vi "INI文件查看器.vi"() -> ()   [LabVIEW 2012, in "Tree Tools.lvlib"]
uses:
  Tree Tools.lvlib
  Core Class/Tree Class/Tree Class.lvclass
  <vilib>/Utility/config.llb/Read Key (String).vi
  <vilib>/Utility/config.llb/NI_LVConfig.lvlib
panel:
  in  "Ini文件":path
  in  "树形":string(tree)
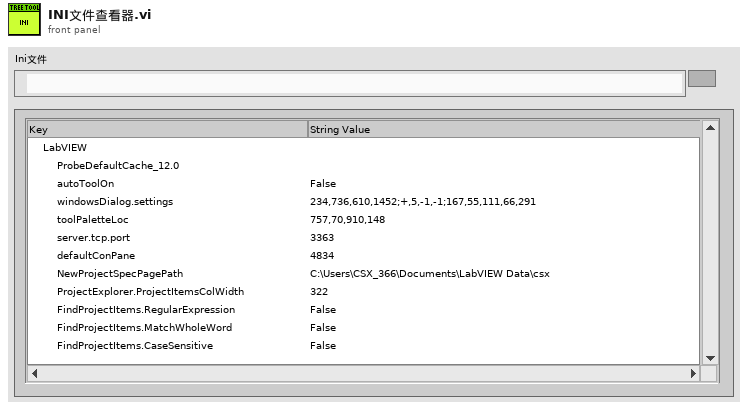
[diagram p1: front panel]
types:
  T1 = typedef "NI_LVConfig.lvlib/Config Data RefNum.ctl" = refnum<k1>
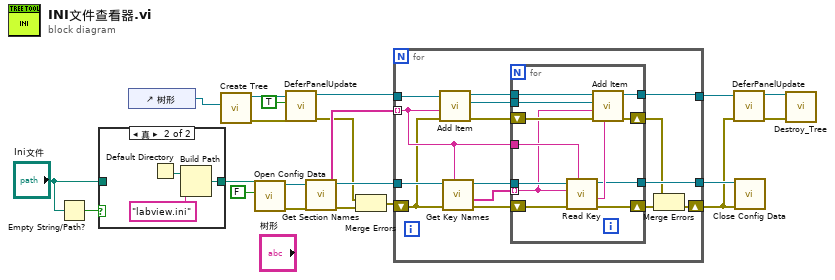
[diagram p0: block diagram]
diagram:
  n1 = Empty String/Path?(string/path="Ini文件") -> (empty?=w6:bool)
  n2 = case shown="真" w6 {
    tunnel: [w22 w23] -> w21
    tunnel: "Ini文件" -> [w22 _]
    frame False {
    }
    frame True {
      n3 = Default Directory() -> (w25:path)
      n4 = Build Path(base path=w25, name or relative path="labview.ini" ("名称或相对路径")) -> (appended path=w23:path)
    }
  }
  n5 = control-ref of="树形"() -> (w17:refnum<vi>)
  n6 = call "Create Tree.vi"("Tree Refnum"=w17) -> ("error out"=w13:errorcluster, "Tree_LVOOP out"=w14:refnum<class "Tree Class.lvclass">)  [unwired: 9 in]
  n7 = call <vilib>:"Open Config Data.vi"("create file if necessary (T)"=FALSE, "configuration file path"=w21) -> ("error out"=w18:errorcluster, "refnum"=w19:T1)  [unwired: 7 in, 1 out]
  n8 = call-dynamic "DeferPanelUpdate.vi"("error in (no error)"=w13, "Defer? (F)"=TRUE, "Tree_LVOOP__lava_lib_tree_class in"=w14) -> ("error out"=w3:errorcluster, "Tree_LVOOP__lava_lib_tree_class out"=w11:refnum<class "Tree Class.lvclass">)  [unwired: 7 in]
  n9 = call <vilib>:"Get Section Names.vi"("error in (no error)"=w18, "refnum"=w19) -> ("error out"=w4:errorcluster, "section names"=w16:string[], "refnum out"=w15:T1)  [unwired: 7 in]
  n10 = Merge Errors(w3, w4) -> (w2:errorcluster)
  n11 = for {
    tunnel: w16 -> [w33] mode=indexing
    tunnel: w15 -> [w39]
    tunnel: [w30] -> w7
    shift-right: [w27] -> w1
    shift-left: w2 -> [w29]
    tunnel: w11 -> [w40]
    tunnel: [w36] -> w10
    n12 = call-dynamic "Add Item.vi"("error in (no error)"=w29, "Text"=w33, "Tree_LVOOP in"=w40) -> ("error out"=w35:errorcluster, "Upmost Created Tag"=w32:refnum<class "Tree Tag Class.lvclass">, "Tree_LVOOP out"=w37:refnum<class "Tree Class.lvclass">)  [unwired: 6 in]
    n13 = call <vilib>:"Get Key Names.vi"("section"=w33, "error in (no error)"=w29, "refnum"=w39) -> ("error out"=w31:errorcluster, "key names"=w38:string[], "refnum out"=w34:T1)  [unwired: 5 in, 1 out]
    n14 = for {
      tunnel: w38 -> [w46] mode=indexing
      shift-right: [w49] -> w26
      shift-left: w35 -> [w50]
      tunnel: w34 -> [w48]
      tunnel: w33 -> [w47]
      tunnel: w32 -> [w44]
      shift-right: [w42] -> w28
      shift-left: w31 -> [w43]
      tunnel: [w41] -> w30
      tunnel: w37 -> [w52]
      tunnel: [w51] -> w36
      n15 = call-poly <vilib>:"Read Key.vi"("section"=w47, "error in (no error)"=w43, "key"=w46, "refnum"=w48) -> ("error out"=w42:errorcluster, "value"=w45:string, "refnum out"=w41:T1)  [unwired: 4 in, 1 out]
      n16 = call-dynamic "Add Item.vi"("Data"=w45, "error in (no error)"=w50, "Text"=w46, "Parent Tag"=w44, "Tree_LVOOP in"=w52) -> ("error out"=w49:errorcluster, "Tree_LVOOP out"=w51:refnum<class "Tree Class.lvclass">)  [unwired: 4 in, 1 out]
    }
    n17 = Merge Errors(w26, w28) -> (w27:errorcluster)
  }
  n18 = call-dynamic "DeferPanelUpdate.vi"("error in (no error)"=w1, "Tree_LVOOP__lava_lib_tree_class in"=w10) -> ("error out"=w8:errorcluster, "Tree_LVOOP__lava_lib_tree_class out"=w9:refnum<class "Tree Class.lvclass">)  [unwired: 8 in]
  n19 = call <vilib>:"Close Config Data.vi"("error in (no error)"=w1, "refnum"=w7) -> ()  [unwired: 8 in, 2 out]
  n20 = call-dynamic "Destroy_Tree.vi"("error in (no error)"=w8, "Tree_LVOOP in"=w9) -> ()  [unwired: 9 in, 1 out]
